vi "Set Visible Plot.vi"(7 "number of plots":i32=-1, 8 "error in (no error)":errorcluster, 10 "Plot Id":i32, 11 "XYGraph in":refnum<vi>) -> (0 "error out":errorcluster)   [LabVIEW 2022 SP3, in "Stepped Frequency Sweep_Class D Amplifier_UI.lvlib"]
uses:
  Stepped Frequency Sweep_Class D Amplifier_UI.lvlib
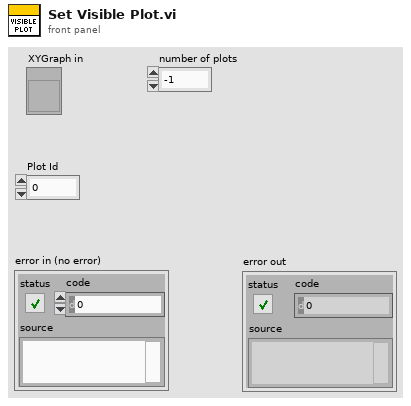
[diagram p1: front panel]
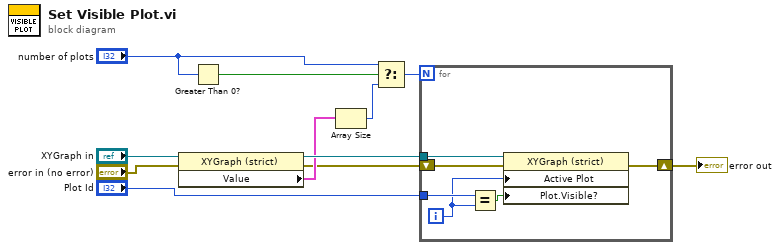
[diagram p0: block diagram]
diagram:
  n1 = property class="XYGraph (strict)"(reference="XYGraph in", error in="error in (no error)") -> (reference out=w10:refnum<vi>, error out=w6:errorcluster, "Value"=w8:cluster{"frequency (Hz)":dbl[], "THD+N":dbl[]}[])
  n2 = Greater Than 0?(x="number of plots") -> (x > 0?=w4:bool)
  n3 = Array Size(array=w8) -> (size(s)=w2:i32)
  n4 = Select(t="number of plots", s=w4, f=w2) -> (s? t:f=w3:i32)
  n5 = for {
    N: w3 -> [_]
    tunnel: w10 -> [w17]
    tunnel: "Plot Id" -> [w16]
    shift-right: [w12] -> w5
    shift-left: w6 -> [w13]
    i -> [w15]
    n6 = Equal?(x=w16, y=w15) -> (x = y?=w14:bool)
    n7 = property class="XYGraph (strict)"(reference=w17, error in=w13, "Active Plot"=w15, "Plot.Visible?"=w14) -> (error out=w12:errorcluster)  [unwired: 1 out]
  }
  "error out" <- w5
